vi "checkConnectionError.vi"(8 "error in (no error)":errorcluster, 11 "TCPClient in":refnum<class "TCPClient.lvclass">) -> (0 "error out":errorcluster, 2 "ConnectionError?":bool, 3 "TCPClient out":refnum<class "TCPClient.lvclass">)   [LabVIEW 2016, in "tcp.lvlib" / "TCPClient.lvclass"]
uses:
  TCPClient.lvclass
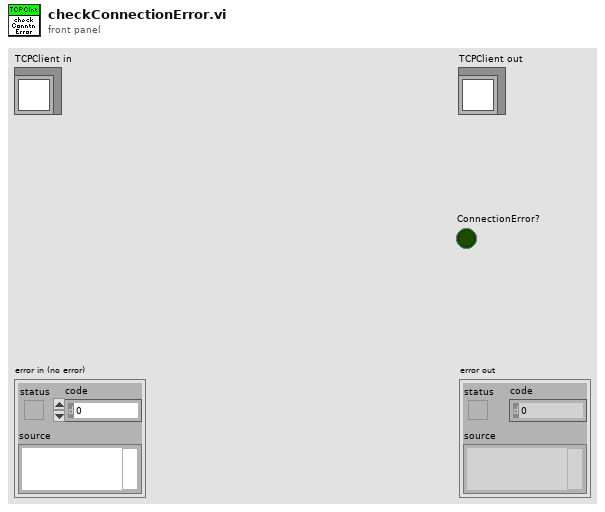
[diagram p1: front panel]
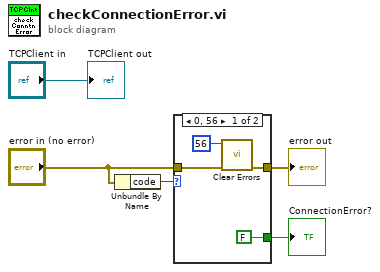
[diagram p0: block diagram]
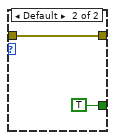
[diagram p2: hidden frame]
diagram:
  n1 = Unbundle By Name("error in (no error)") -> ("code"=w1:i32)
  n2 = case shown="0, 56" w1 {
    tunnel: [w7 w10] -> w4
    tunnel: [FALSE ("ConnectionError?") TRUE ("ConnectionError?")] -> w3
    tunnel: "error in (no error)" -> [w8 w10]
    frame 0, 56 {
      n3 = call <vilib>:"Clear Errors.vi"("error in (no error)"=w8, "specific error code to clear (0: all)"=56) -> ("error out"=w7:errorcluster)  [unwired: 4 in, 1 out]
    }
    frame Default {
    }
  }
  "error out" <- w4
  "ConnectionError?" <- w3
  "TCPClient out" <- "TCPClient in"
